vi "Stepper_Motor.vi"() -> ()   [LabVIEW 2009]
uses:
  <vilib>/DAQmx/configure/timing.llb/DAQmx Timing (Sample Clock).vi
  <vilib>/Waveform/DWDTOps.llb/DWDT Analog to Digital.vi
  <vilib>/DAQmx/create/channels.llb/DAQmx Create Channel (DO-Digital Output).vi
  <vilib>/DAQmx/write.llb/DAQmx Write (Digital Wfm 1Chan NSamp).vi
panel:
  out "error out":errorcluster
  in  "stop":bool
  out "Waveform Graph":waveform(i32)(graph)
  in  "sample frequency":dbl
  in  "frequency":dbl
  in  "Amplitude":dbl
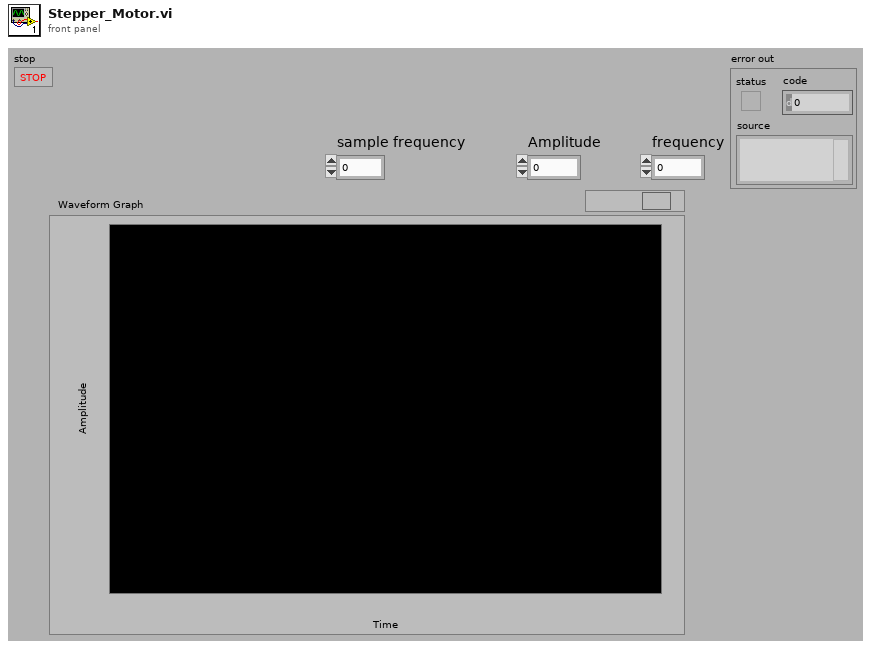
[diagram p1: front panel]
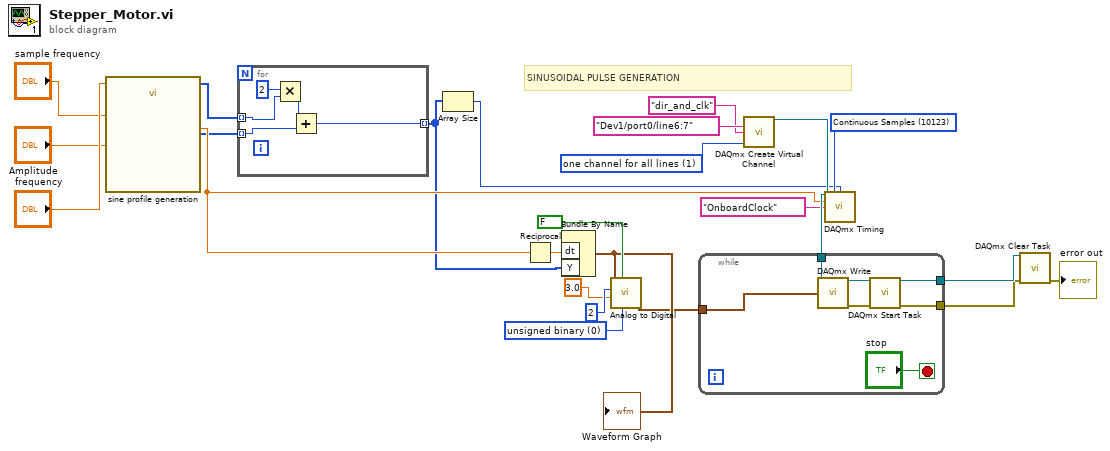
[diagram p0: block diagram]
diagram:
  w10 = u16 0 items=["unsigned binary", "offset binary", "2's complement"] ("data format (offset binary)")
  w21 = 10123 items=["Finite Samples"=10178, "Continuous Samples"=10123, "Hardware Timed Single Point"=12522] ("sample mode")
  w16 = 1 items=["one channel for each line", "one channel for all lines"] ("line grouping")
  # "SINUSOIDAL PULSE GENERATION"
  n1 = call "sine profile generation.vi"("frequency"="frequency", "amplitude in degrees"="Amplitude", "sample frequency"="sample frequency") -> ("sample frequency 2"=w13:dbl, "Direction Pulse Array"=w2:i16[], "Clock Pulse Array"=w1:i32[])  [unwired: 5 out]
  n2 = for {
    tunnel: w2 -> [w28] mode=indexing
    tunnel: w1 -> [w26] mode=indexing
    tunnel: [w29] -> w9 mode=indexing
    n3 = Multiply(x=i16 2, y=w28) -> (x*y=w30:i16)
    n4 = Add(x=w30, y=w26) -> (x+y=w29:i32)
  }
  n5 = Array Size(array=w9) -> (size(s)=w8:i32)
  n6 = Reciprocal(x=w13) -> (1/x=w17:dbl)
  n7 = Bundle By Name("dt"=w17, "Y"=w9) -> (w7:waveform(i32))  [unwired: 1 in]
  "Waveform Graph" <- w7
  n8 = call-poly <vilib>:"Analog to Digital.vi"("data format (offset binary)"=w10, "compress digital (T)"=FALSE, "full-scale range (pk-pk)"=3.0, "resolution (16 bit)"=2, "analog waveform"=w7) -> ("digital waveform"=w6:digitalwaveform)  [unwired: 3 in, 3 out]
  n9 = call-poly <vilib>:"DAQmx Create Virtual Channel.vi"("lines"=tag "Dev1/port0/line6:7", "name to assign"="dir_and_clk", "line grouping"=w16) -> ("task out"=w20:refnum<k21>)  [unwired: 11 in, 1 out]
  n10 = call-poly <vilib>:"DAQmx Timing.vi"("task/channels in"=w20, "sample mode"=w21, "samples per channel"=w8, "rate"=w13, "source"=tag "OnboardClock") -> ("task out"=w22:refnum<k21>)  [unwired: 9 in, 1 out]
  n11 = while {
    tunnel: w22 -> [w36]
    tunnel: w6 -> [w35]
    tunnel: [w33] -> w5
    tunnel: [w32] -> w4
    stop <- "stop" stop-if-true
    n12 = call-poly <vilib>:"DAQmx Write.vi"("task/channels in"=w36, "data"=w35) -> ("task out"=w37:refnum<k21>, "error out"=w31:errorcluster)  [unwired: 11 in, 1 out]
    n13 = call <vilib>:"DAQmx Start Task.vi"("task/channels in"=w37, "error in"=w31) -> ("task out"=w33:refnum<k21>, "error out"=w32:errorcluster)  [unwired: 12 in]
  }
  n14 = call <vilib>:"DAQmx Clear Task.vi"("task in"=w5, "error in"=w4) -> ("error out"=→"error out":errorcluster)  [unwired: 13 in]
